vi "PreProcess.vi"(8 "error in (no error)":errorcluster, 9 "Input array":sgl[](array[numeric]), 10 "Variant in":variant, 11 "ONNX Class in":refnum<class "ONNX Class.lvclass">) -> (0 "error out":errorcluster, 2 "Variant out":variant, 3 "ONNX Class out":refnum<class "ONNX Class.lvclass">)   [LabVIEW 2018, in "ONNX Class Library.lvlib" / "ONNX Class.lvclass"]
uses:
  ONNX Class.lvclass
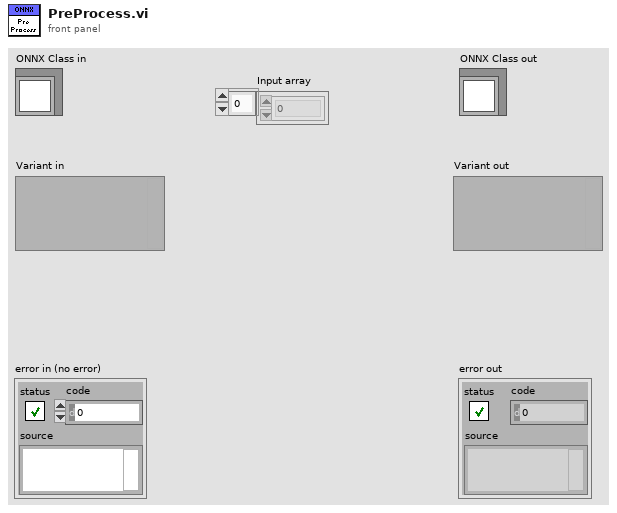
[diagram p1: front panel]
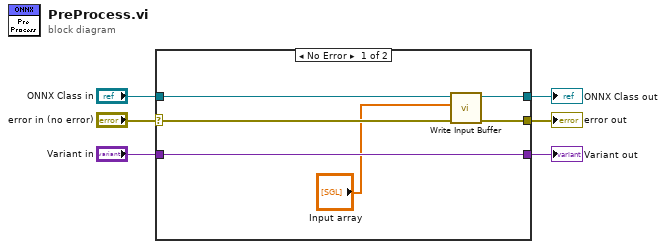
[diagram p0: block diagram]
diagram:
  n1 = case shown="No Error" "error in (no error)" {
    selector: "error in (no error)" -> [w9 w15]
    tunnel: [w8 w15] -> w5
    tunnel: [w10 w14] -> w3
    tunnel: "ONNX Class in" -> [w11 w14]
    tunnel: "Variant in" -> [w12 w13]
    tunnel: [w12 w13] -> w1
    frame No Error {
      n2 = call-dynamic "Write Input Buffer.vi"("error in (no error)"=w9, "Input Buffer"="Input array", "ONNX Class in"=w11) -> ("error out"=w8:errorcluster, "ONNX Class out"=w10:refnum<class "ONNX Class.lvclass">)  [unwired: 7 in]
    }
    frame Error {
    }
  }
  "error out" <- w5
  "ONNX Class out" <- w3
  "Variant out" <- w1
